vi "ToRepo.vi"(8 "error in":errorcluster, 9 "to repo cluster":T1, 10 "repository in":refnum<class "NISE_CEF_Repository.lvclass">, 11 "cRIO in":refnum<class "_cRIO.lvclass">) -> (0 "error out":errorcluster, 2 "repository out":refnum<class "NISE_CEF_Repository.lvclass">, 3 "cRIO out":refnum<class "_cRIO.lvclass">)   [LabVIEW 2013, in "_cRIO.lvclass"]
uses:
  _cRIO.lvclass
  CEF_TreeControl/Repository/NISE_CEF_Repository.lvclass
  CEF_TreeControl/Node/ToRepoCluster.ctl
  cRIO Repo/_cRIORepo.lvclass
  cRIO Repo/ChannelData.ctl
  _cRIO.lvclass/_cRIO.ctl
  CEF_TreeControl/Node/NISE_CEF_Node.lvclass
  cRIO Repo/_cRIORepo.lvclass/_cRIORepo.ctl
  Read System Name.vi
  cRIO Repo/Write System.vi
  cRIO Repo/Write Channels.vi
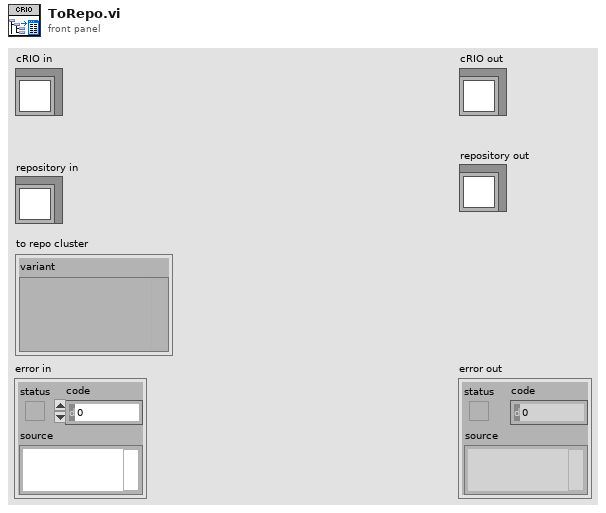
[diagram p1: front panel]
types:
  T1 = typedef "NISE_CEF_Node.lvclass/ToRepoCluster.ctl" = cluster{"variant":variant}
  T2 = typedef "_cRIORepo.lvclass/ChannelData.ctl" = cluster{"channel group":string, "channel name":string, "IO ":string, "sensor ID":string, "description":string, "system":string, "channel type":string}
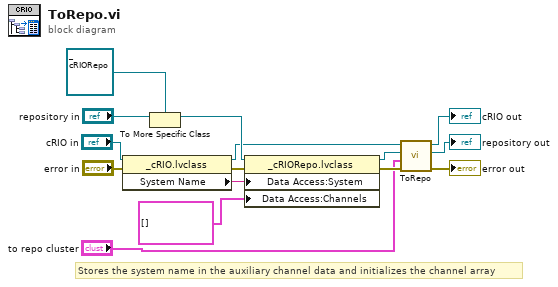
[diagram p0: block diagram]
diagram:
  # "Stores the system name in the auxiliary channel data and initializes the channel array"
  n1 = property class="_cRIO.lvclass"(reference="cRIO in", error in="error in") -> (reference out=w6:refnum<class "_cRIO.lvclass">, error out=w4:errorcluster, "System Name"=w8:string)
  n2 = To More Specific Class(target class=refnum<class "_cRIORepo.lvclass"> refnum ("cRIO repo.lvclass"), reference="repository in") -> (specific class reference=w9:refnum<class "_cRIORepo.lvclass">)  [unwired: 1 in, 1 out]
  n3 = property class="_cRIORepo.lvclass"(reference=w9, error in=w4, "Data Access:System"=w8, "Data Access:Channels"=T2[] [] ("channels")) -> (reference out=w12:refnum<class "_cRIORepo.lvclass">, error out=w3:errorcluster)
  n4 = call-parent "ToRepo.vi"("error in"=w3, "to repo cluster"="to repo cluster", "repository in"=w12, "node in"=w6) -> ("error out"=→"error out":errorcluster, "repository out"=→"repository out":refnum<class "NISE_CEF_Repository.lvclass">, "node out"=→"cRIO out":refnum<class "_cRIO.lvclass">)  [unwired: 5 in]
